vi "Page_Advanced_Quit.vi"(6 "ctl references":T1, 8 "error in (no error)":errorcluster, 9 "data":variant, 10 "Target":refnum<vi>, 11 "AB_Application in":refnum<class "AB_Application.lvclass">) -> (0 "error out":errorcluster, 3 "AB_Application out":refnum<class "AB_Application.lvclass">)   [LabVIEW 2020, in "AB_Application.lvclass"]
uses:
  <vilib>/AppBuilder/AB_Classes/Application/AB_Application.lvclass
  <vilib>/AppBuilder/AB_Classes/Application/AB_Application.lvclass/AB_Application.ctl
  <resource>/Framework/Providers/Builds/AppBuilder/AB_UI_Page_Advanced_References.ctl
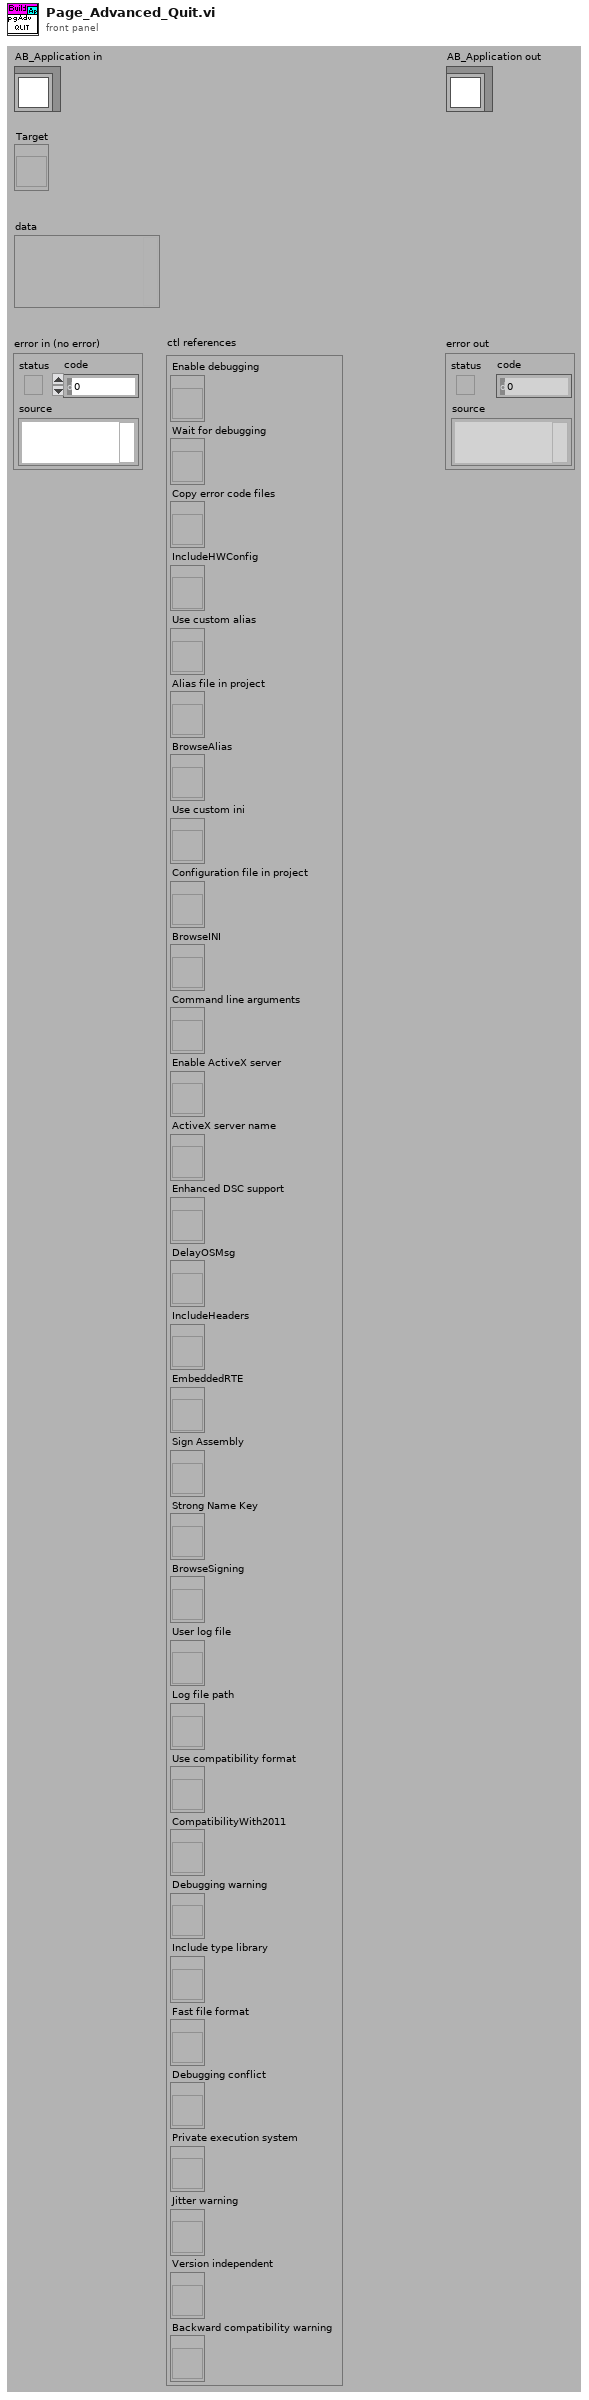
[diagram p1: front panel]
types:
  T1 = typedef "AB_UI_Page_Advanced_References.ctl" = cluster{"Enable debugging":refnum<vi>, "Wait for debugging":refnum<vi>, "Copy error code files":refnum<vi>, "IncludeHWConfig":refnum<vi>, "Use custom alias":refnum<vi>, "Alias file in project":refnum<vi>, "BrowseAlias":refnum<vi>, "Use custom ini":refnum<vi>, "Configuration file in project":refnum<vi>, "BrowseINI":refnum<vi>, "Command line arguments":refnum<vi>, "Enable ActiveX server":refnum<vi>, "ActiveX server name":refnum<vi>, "Enhanced DSC support":refnum<vi>, "DelayOSMsg":refnum<vi>, "IncludeHeaders":refnum<vi>, "EmbeddedRTE":refnum<vi>, "Sign Assembly":refnum<vi>, "Strong Name Key":refnum<vi>, "BrowseSigning":refnum<vi>, "User log file":refnum<vi>, "Log file path":refnum<vi>, "Use compatibility format":refnum<vi>, "CompatibilityWith2011":refnum<vi>, "Debugging warning":refnum<vi>, "Include type library":refnum<vi>, "Fast file format":refnum<vi>, "Debugging conflict":refnum<vi>, "Private execution system":refnum<vi>, "Jitter warning":refnum<vi>, "Version independent":refnum<vi>, "Backward compatibility warning":refnum<vi>}
  T2 = typedef "AB_Application.ctl" = cluster{"INI_path":path, "INI_itemID":string, "INI_GUID":string, "aliasPath":path, "aliasItemID":string, "aliasGUID":string, "waitDebugging":bool, "copyErrors":bool, "useFFRTE":bool, "includeHWConfig":bool, "showHWConfig":bool, "winsec.certificate":string, "winsec.timestamp":string, "winsec.description":string, "winsec.manifestItemID":string, "winsec.manifestPath":path, "web service itemIDs":string[], "Embedded Server Configuration":T3, "Server Type":enum32{"NI Web Server", "Application Web Server"}}
  T3 = typedef "AB_Embedded_Server_Configuration.ctl" = cluster{"HTTP enabled?":bool, "HTTP port":i32, "HTTPS enabled?":bool, "HTTPS port":i32, "SSL certificate file":path}
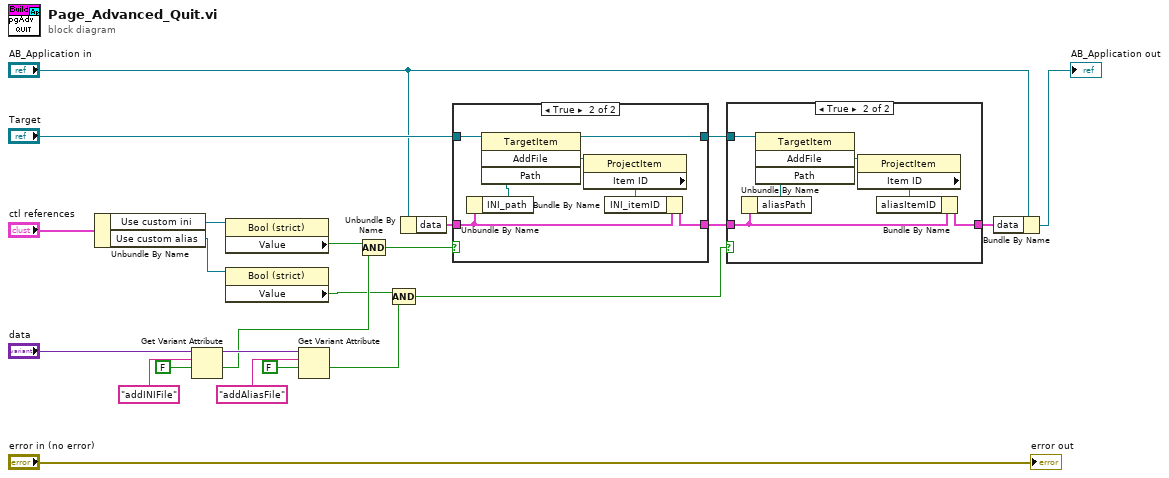
[diagram p0: block diagram]
diagram:
  n1 = Unbundle By Name("ctl references") -> ("Use custom ini"=w15:refnum<vi>, "Use custom alias"=w12:refnum<vi>)
  n2 = Get Variant Attribute(Variant="data", name="addINIFile", default value (empty Variant)=FALSE) -> (duplicate Variant=w22:variant, value=w13:bool)  [unwired: 1 in, 2 out]
  n3 = property class="Bool (strict)"(reference=w15) -> ("Value"=w14:bool)  [unwired: 1 in, 2 out]
  n4 = property class="Bool (strict)"(reference=w12) -> ("Value"=w11:bool)  [unwired: 1 in, 2 out]
  n5 = Get Variant Attribute(Variant=w22, name="addAliasFile", default value (empty Variant)=FALSE) -> (value=w10:bool)  [unwired: 1 in, 3 out]
  n6 = Compound Arithmetic op=AND(w14, w13) -> (w6:bool)
  n7 = Compound Arithmetic op=AND(w11, w10) -> (w5:bool)
  n8 = Unbundle By Name("AB_Application in") -> ("data"=w4:T2)
  n9 = case shown="True" w6 {
    tunnel: "Target" -> [w25 w31]
    tunnel: [w25 w30] -> w9
    tunnel: w4 -> [w24 w28]
    tunnel: [w24 w26] -> w8
    frame False {
    }
    frame True {
      n10 = Unbundle By Name(w28) -> ("INI_path"=w29:path)
      n11 = invoke class="TargetItem" method="AddFile"(reference=w31, "Path"=w29) -> (reference out=w30:refnum<vi>, "AddFile"=w32:refnum<vi>)  [unwired: 2 in, 2 out]
      n12 = property class="ProjectItem"(reference=w32) -> ("Item ID"=w27:string)  [unwired: 1 in, 2 out]
      n13 = Bundle By Name(cluster=w28, "INI_itemID"=w27) -> (w26:T2)
    }
  }
  n14 = case shown="True" w5 {
    tunnel: w9 -> [_ w38]
    tunnel: [w33 w36] -> w3
    tunnel: w8 -> [w33 w37]
    frame False {
    }
    frame True {
      n15 = Unbundle By Name(w37) -> ("aliasPath"=w35:path)
      n16 = invoke class="TargetItem" method="AddFile"(reference=w38, "Path"=w35) -> ("AddFile"=w39:refnum<vi>)  [unwired: 2 in, 3 out]
      n17 = property class="ProjectItem"(reference=w39) -> ("Item ID"=w34:string)  [unwired: 1 in, 2 out]
      n18 = Bundle By Name(cluster=w37, "aliasItemID"=w34) -> (w36:T2)
    }
  }
  n19 = Bundle By Name(cluster="AB_Application in", "data"=w3) -> (→"AB_Application out":refnum<class "AB_Application.lvclass">)
  "error out" <- "error in (no error)"
